vi "Close.vi"(8 "error in (no error)":errorcluster, 11 "Agilent_3458A in":refnum<class "Agilent_3458A.lvclass">) -> (0 "error out":errorcluster, 3 "Agilent_3458A out":refnum<class "Agilent_3458A.lvclass">)   [LabVIEW 2018, in "DigitizerPlugins.lvlib" / "Agilent_3458A.lvclass"]
uses:
  Agilent_3458A.lvclass
  Y:/Projects/PMUCal/Modules/Digitizer/DigitizerPlugins/DigitizerBaseClass/DigitizerBase.lvclass
  DigitizerBaseClass/DigitizerBase.lvclass/DigitizerBase.ctl
  DigitizerBaseClass/Accessors/Read InstRef.vi
  DigitizerBaseClass/Accessors/Write InstRef.vi
  <instrlib>/Agilent 3458/Agilent 3458.lvlib
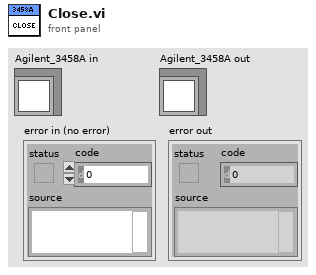
[diagram p1: front panel]
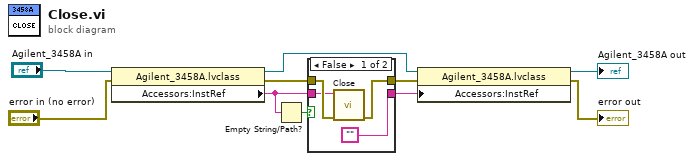
[diagram p0: block diagram]
diagram:
  n1 = property class="Agilent_3458A.lvclass"(reference="Agilent_3458A in", error in="error in (no error)") -> (reference out=w8:refnum<class "Agilent_3458A.lvclass">, error out=w6:errorcluster, "Accessors:InstRef"=w2:string)
  n2 = Empty String/Path?(string/path=w2) -> (empty?=w1:bool)
  n3 = case shown="False" w1 {
    tunnel: ["" w15] -> w7
    tunnel: w6 -> [w13 w16]
    tunnel: [w12 w16] -> w5
    tunnel: w2 -> [w11 w15]
    frame False {
      n4 = call <instrlib>:"Close.vi"("error in (no error)"=w13, "VISA resource name"=w11) -> ("error out"=w12:errorcluster)  [unwired: 9 in]
    }
    frame True {
    }
  }
  n5 = property class="Agilent_3458A.lvclass"(reference=w8, error in=w5, "Accessors:InstRef"=w7) -> (reference out=→"Agilent_3458A out":refnum<class "Agilent_3458A.lvclass">, error out=→"error out":errorcluster)
